vi "L1LeftToCargo7.vi"(9 "Initialized":bool) -> (2 "Drive State":T1)   [LabVIEW 2018]
uses:
  driveStateEnum.ctl
  L1LeftToCargo7.ctl
  driveShifterEnum.ctl
  L1RightToCargo8.ctl
  HatchPanel/hatchPanelEnum.ctl
  HatchPanel/hatchPanelNotifierCluster.ctl
  MotionProfile/Constants.vi
panel:
  out "Speed (ft/s) 3":dbl=5.820510365604576
  in  "Wait til slower then(ft/s) 3":dbl=-3.0
  out "Speed (ft/s) 2":dbl=5.820510365604576
  in  "Wait til slower then(ft/s) 2":dbl=-3.0
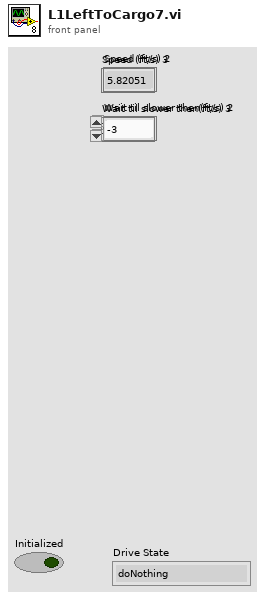
[diagram p1: front panel]
types:
  T1 = typedef "driveStateEnum.ctl" = enum16{"doNothing", "Manuel", "Teleop", "Follow Path (init)", "Follow Path", "Move to Target", "Climb", "Line Align", "Rotate180", "Align50Degrees", "Sonar Brake Tele", "LLCushion", "Auto Approach Target"}
  T2 = typedef "L1LeftToCargo7.ctl" = enum16{"7b -  back away from cargo ship ", "1 - MP move to cargo Ship (init)", "2 - MP move to cargo ship", "3 - Delay for shift", "4 - Approach To Score", "5 - Scored", "99 - doNothing", "7a - back away from cargo ship (init)", "8 - Hatch Panel Motion Off", "9 - Scoring Claw On", "8 - turn towards loading station", "10 - Scoring Claw Off", "11 - MP move towards loading station (init)", "12 -  MP move towards loading station", "13 - MP Move towards  cargo ship *2 (init)", "14 - MP Move towards  cargo ship *2"}
  T3 = typedef "WPI_MotorControlDeviceRef.ctl" = cluster{"DeviceStatus":errorcluster, "Type":T4, "PWM":cluster{"PWM Channel":T5, "DeadBand":T6}, "CAN":cluster{"Device Number":u8, "SetOutput VI Ref":variant, "GetOutput VI Ref":variant, "Enable VI Ref":variant, "Disable VI Ref":variant, "Data":variant}, "Invert":bool, "DIO PWM":cluster{"PWM \"Enable\" Channel":T5, "DIOChannel":T7, "PWM Rate":dbl}}
  T4 = typedef "WPI_MotorControlType.ctl" = enum16{"PWM", "CAN", "DIO PWM"}
  T5 = typedef "FPGA_DIOPWMChannel.ctl" = enum8{"PWM 0", "PWM 1", "PWM 2", "PWM 3", "PWM 4", "PWM 5", "PWM 6", "PWM 7", "PWM 8", "PWM 9", "PWM MXP 0", "PWM MXP 1", "PWM MXP 2", "PWM MXP 3", "PWM MXP 4", "PWM MXP 5", "PWM MXP 6", "PWM MXP 7", "PWM MXP 8", "PWM MXP 9", "Invalid"}
  T6 = typedef "WPI_PWMDeadband.ctl" = cluster{"Name":string, "maxPositivePwm":i32, "minPositivePwm":i32, "centerPwm":i32, "maxNegativePwm":i32, "minNegativePwm":i32, "angularRange":u16}
  T7 = typedef "FPGA_DIOChannel.ctl" = enum8{"DIO 0", "DIO 1", "DIO 2", "DIO 3", "DIO 4", "DIO 5", "DIO 6", "DIO 7", "DIO 8", "DIO 9", "DIO MXP 0", "DIO MXP 1", "DIO MXP 2", "DIO MXP 3", "DIO MXP 4", "DIO MXP 5", "DIO MXP 6", "DIO MXP 7", "DIO MXP 8", "DIO MXP 9", "DIO MXP 10", "DIO MXP 11", "DIO MXP 12", "DIO MXP 13", "DIO MXP 14", "DIO MXP 15", "SPI Port CS1", "SPI Port CS2", "SPI Port CS3", "SPI Port MISO", "SPI Port MOSI", "Invalid"}
  T8 = typedef "L1RightToCargo8.ctl" = enum16{"7b -  back away from cargo ship ", "1 - MP move to cargo Ship (init)", "2 - MP move to cargo ship", "3 - Delay for shift", "4 - Approach To Score", "5 - Scored", "99 - doNothing", "7a - back away from cargo ship (init)", "8 - Hatch Panel Motion Off", "9 - Scoring Claw On", "8 - turn towards loading station", "10 - Scoring Claw Off", "11 - MP move towards loading station (init)", "12 -  MP move towards loading station", "13 - MP Move towards  cargo ship *2 (init)", "14 - MP Move towards  cargo ship *2"}
  T9 = typedef "driveShifterEnum.ctl" = enum16{"Low", "High"}
  T10 = typedef "hatchPanelNotifierCluster.ctl" = cluster{"Hatch Panel State":T11, "Mechanism Motion":bool, "Gathering Claw Motion":bool, "Scoring Claw Motion":bool}
  T11 = typedef "hatchPanelEnum.ctl" = enum16{"do nothing", "State Machine", "Stach Mode", "Climb Mode", "Retracted Closed", "Retracted Open", "Extended Closed", "Extended Open"}
  T12 = typedef "CTRE_PigeonIMU_DeviceRef.ctl" = cluster{"DeviceStatus":errorcluster, "Device Number":u8, "Type":T13, "Device ID":u32, "Handle":u64, "UsageFrame":u32, "Library Path":path}
  T13 = typedef "CTRE_PigeonIMU_ConnectionType.ctl" = u32
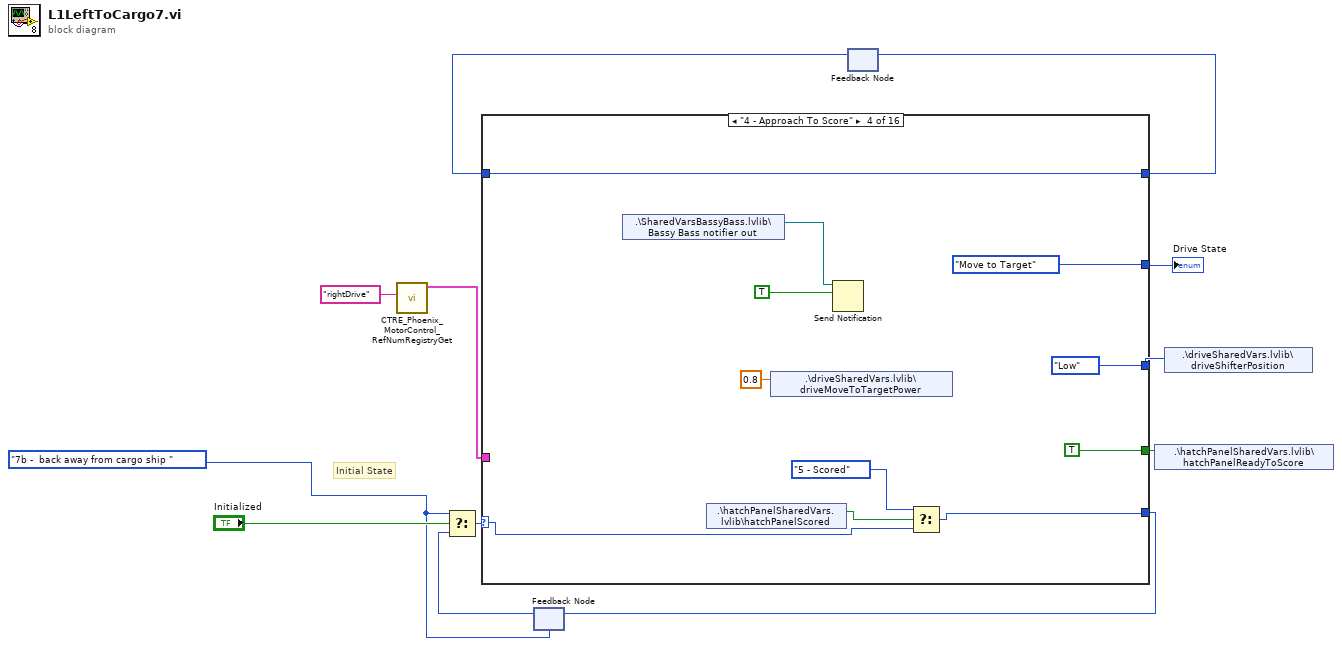
[diagram p0: block diagram]
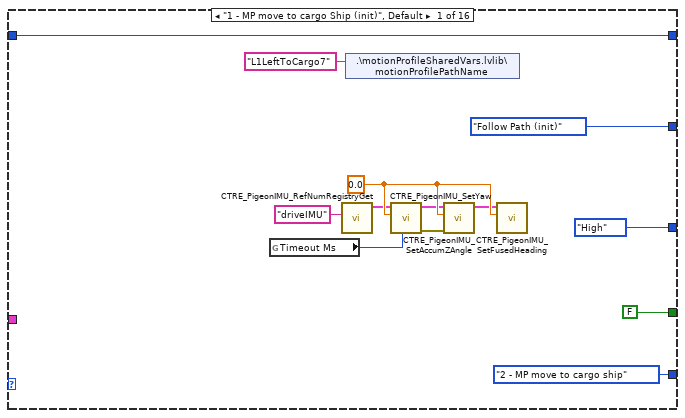
[diagram p2: hidden frame]
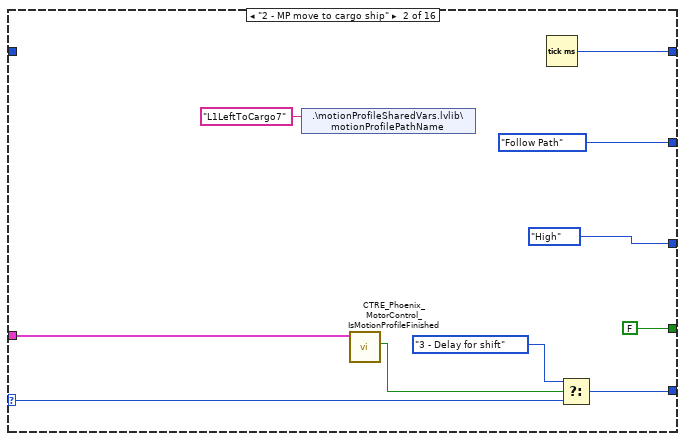
[diagram p3: hidden frame]
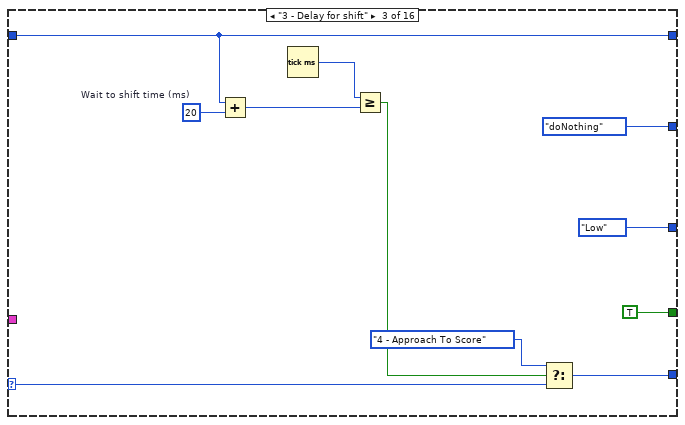
[diagram p4: hidden frame]
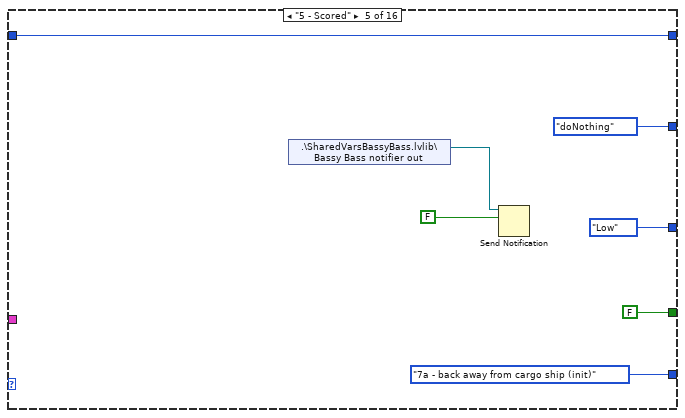
[diagram p5: hidden frame]
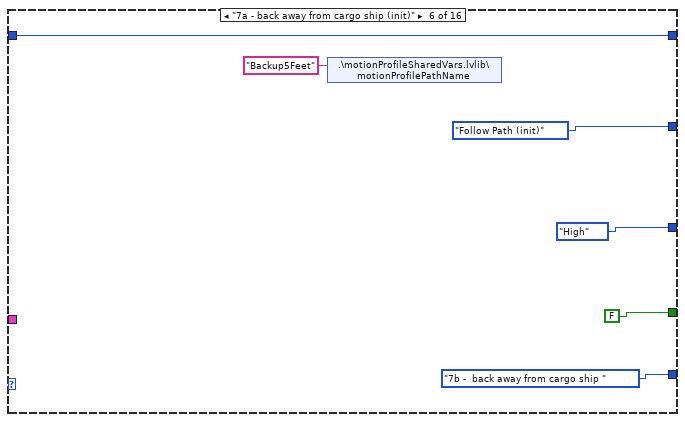
[diagram p6: hidden frame]
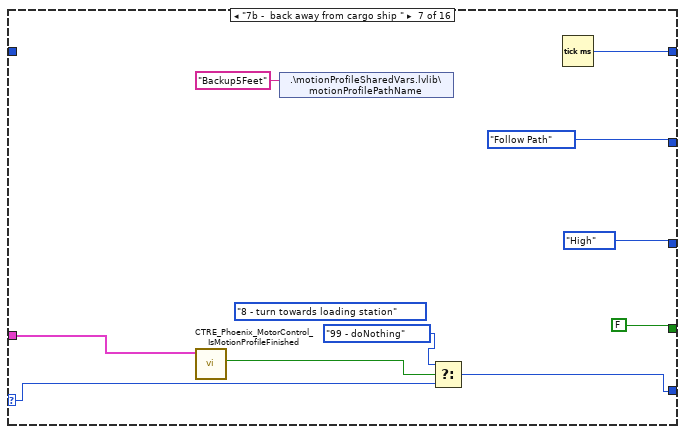
[diagram p7: hidden frame]
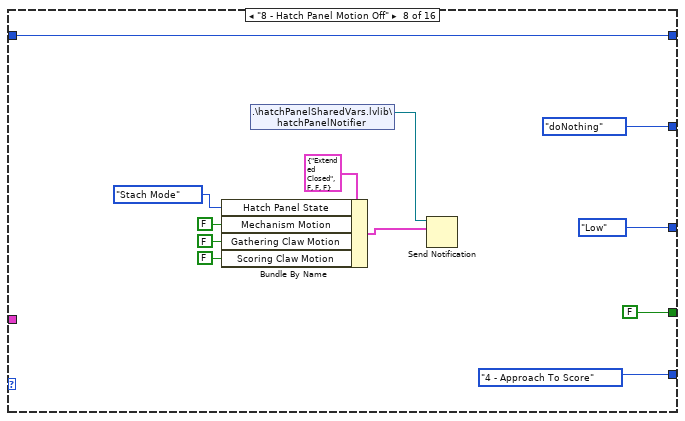
[diagram p8: hidden frame]
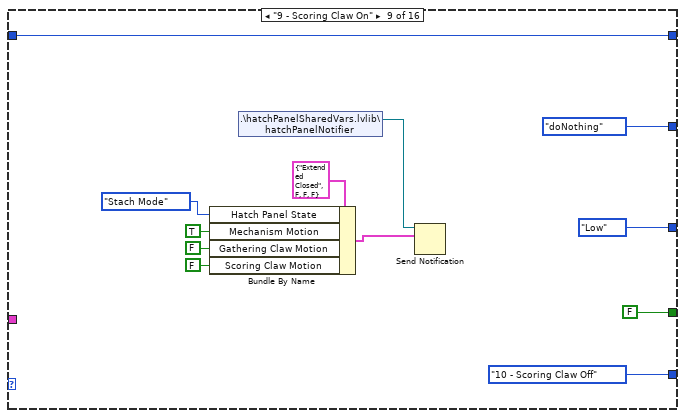
[diagram p9: hidden frame]
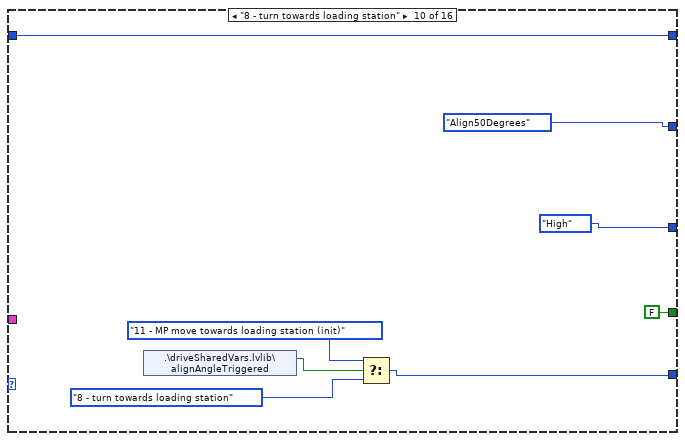
[diagram p10: hidden frame]
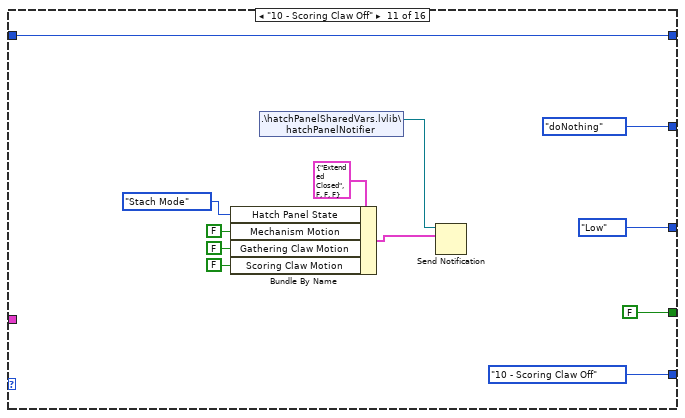
[diagram p11: hidden frame]
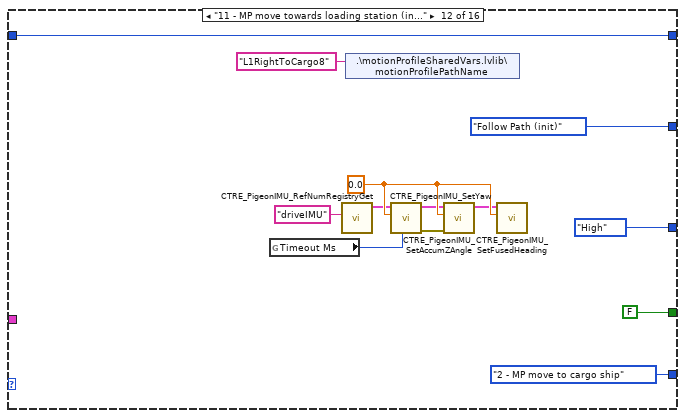
[diagram p12: hidden frame]
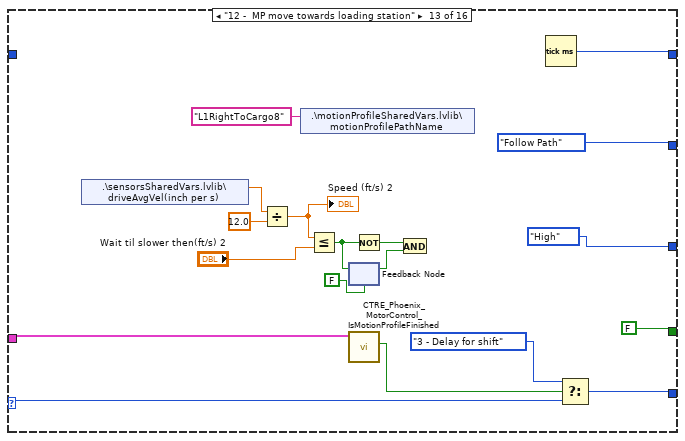
[diagram p13: hidden frame]
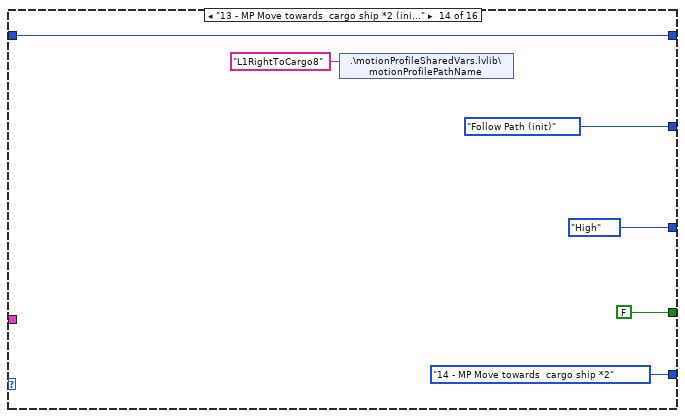
[diagram p14: hidden frame]
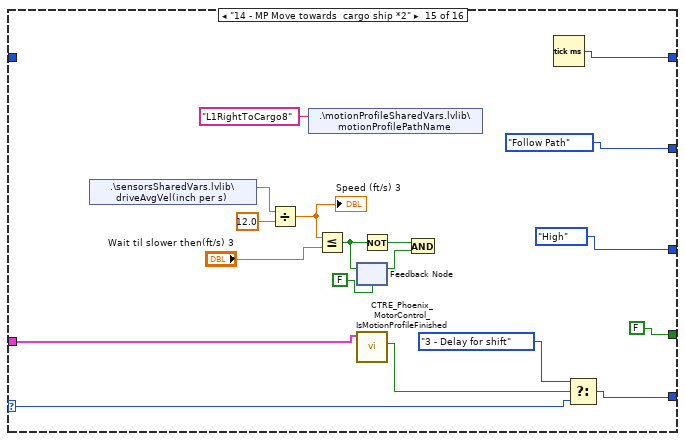
[diagram p15: hidden frame]
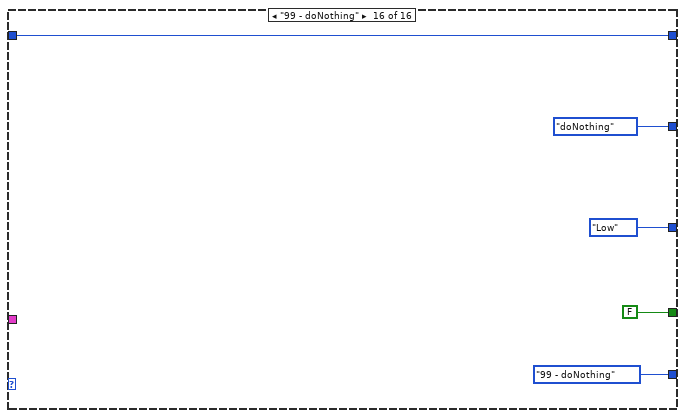
[diagram p16: hidden frame]
diagram:
  w1 = L1LeftToCargo7."7b -  back away from cargo ship " ("Enum")
  # "Initial State"
  n1 = call <vilib>:"CTRE_Phoenix_MotorControl_RefNumRegistryGet.vi"("refnum name"="rightDrive") -> ("PhoenixMotorControlDevRef"=w8:T3)  [unwired: 9 in, 1 out]
  n2 = feedback #1(w1) -> (w11:T8)
  n3 = Select(t=w1, s="Initialized", f=w11) -> (s? t:f=w12:T8)
  n4 = feedback #2() -> (w3:u32)  [unwired: 1 in]
  n5 = case shown="\"4 - Approach To Score\"" w12 {
    selector: w12 -> [_ w33 w38 w51 _ _ w73 _ _ _ _ _ w143 _ w168 _]
    tunnel: [L1RightToCargo8."2 - MP move to cargo ship" ("Enum") w34 w40 w50 L1RightToCargo8."7a - back away from cargo ship (init)" ("Enum") L1RightToCargo8."7b -  back away from cargo ship " ("Enum") w72 L1RightToCargo8."4 - Approach To Score" ("Enum") L1RightToCargo8."10 - Scoring Claw Off" ("Enum") w105 L1RightToCargo8."10 - Scoring Claw Off" ("Enum") L1RightToCargo8."2 - MP move to cargo ship" ("Enum") w144 L1RightToCargo8."14 - MP Move towards  cargo ship *2" ("Enum") w167 L1RightToCargo8."99 - doNothing" ("Enum")] -> w10
    tunnel: [driveStateEnum."Follow Path (init)" ("Drive State Enum") driveStateEnum."Follow Path" ("Drive State Enum") driveStateEnum."doNothing" ("Drive State Enum") driveStateEnum."Move to Target" ("Drive State Enum") driveStateEnum."doNothing" ("Drive State Enum") driveStateEnum."Follow Path (init)" ("Drive State Enum") driveStateEnum."Follow Path" ("Drive State Enum") driveStateEnum."doNothing" ("Drive State Enum") driveStateEnum."doNothing" ("Drive State Enum") driveStateEnum."Align50Degrees" ("Drive State Enum") driveStateEnum."doNothing" ("Drive State Enum") driveStateEnum."Follow Path (init)" ("Drive State Enum") driveStateEnum."Follow Path" ("Drive State Enum") driveStateEnum."Follow Path (init)" ("Drive State Enum") driveStateEnum."Follow Path" ("Drive State Enum") driveStateEnum."doNothing" ("Drive State Enum")] -> w6
    tunnel: w8 -> [_ w31 _ _ _ _ w74 _ _ _ _ _ w142 _ w162 _]
    tunnel: [driveShifterEnum."High" ("driveShifterPosition") driveShifterEnum."High" ("driveShifterPosition") driveShifterEnum."Low" ("driveShifterPosition") driveShifterEnum."Low" ("driveShifterPosition") driveShifterEnum."Low" ("driveShifterPosition") driveShifterEnum."High" ("driveShifterPosition") driveShifterEnum."High" ("driveShifterPosition") driveShifterEnum."Low" ("driveShifterPosition") driveShifterEnum."Low" ("driveShifterPosition") driveShifterEnum."High" ("driveShifterPosition") driveShifterEnum."Low" ("driveShifterPosition") driveShifterEnum."High" ("driveShifterPosition") driveShifterEnum."High" ("driveShifterPosition") driveShifterEnum."High" ("driveShifterPosition") driveShifterEnum."High" ("driveShifterPosition") driveShifterEnum."Low" ("driveShifterPosition")] -> w5
    tunnel: [w15 w28 w44 w55 w60 w69 w75 w85 w97 w111 w114 w126 w139 w160 w163 w180] -> w4
    tunnel: w3 -> [w15 _ w44 w55 w60 w69 _ w85 w97 w111 w114 w126 _ w160 _ w180]
    tunnel: [FALSE FALSE TRUE TRUE FALSE FALSE FALSE FALSE FALSE FALSE FALSE FALSE FALSE FALSE FALSE FALSE] -> w2
    frame "1 - MP move to cargo Ship (init)", Default {
      w23 = 0.0 ("Angle (Deg)")
      n6 = global read "Constants.vi" "Timeout Ms"() -> (w20:i32)
      n7 = call <vilib>:"CTRE_PigeonIMU_RefNumRegistryGet.vi"("refnum name"="driveIMU") -> ("PigeonIMUDevRef"=w17:T12)  [unwired: 9 in, 1 out]
      n8 = shared-variable ".\\motionProfileSharedVars.lvlib\\motionProfilePathName"("L1LeftToCargo7" ("motionProfilePathName")) -> ()  [unwired: 1 in, 1 out]
      n9 = call <vilib>:"CTRE_PigeonIMU_SetYaw.vi"("timeoutMs"=w20, "Value"=w23, "PigeonIMUDevRef"=w17) -> ("error out"=w18:errorcluster, "PigeonIMUDevRef"=w19:T12)  [unwired: 7 in]
      n10 = call <vilib>:"CTRE_PigeonIMU_SetAccumZAngle.vi"("error in (no error)"=w18, "Angle (Deg)"=w23, "PigeonIMUDevRef"=w19) -> ("PigeonIMUDevRef"=w21:T12)  [unwired: 7 in, 1 out]
      n11 = call <vilib>:"CTRE_PigeonIMU_SetFusedHeading.vi"("Value"=w23, "PigeonIMUDevRef 2"=w21) -> ()  [unwired: 8 in, 2 out]
    }
    frame "2 - MP move to cargo ship" {
      n12 = shared-variable ".\\motionProfileSharedVars.lvlib\\motionProfilePathName"("L1LeftToCargo7" ("motionProfilePathName")) -> ()  [unwired: 1 in, 1 out]
      n13 = call <vilib>:"CTRE_Phoenix_MotorControl_IsMotionProfileFinished.vi"("PhoenixMotorControlDevRef"=w31) -> ("Is Motion Profile Finished?"=w30:bool)  [unwired: 8 in, 2 out]
      n14 = Tick Count (ms)() -> (millisecond timer value=w28:u32)
      n15 = Select(t=L1RightToCargo8."3 - Delay for shift", s=w30, f=w33) -> (s? t:f=w34:T8)
    }
    frame "3 - Delay for shift" {
      w43 = u32 20  # Wait to shift time (ms)
      n16 = Add(x=w44, y=w43) -> (x+y=w41:u32)
      n17 = Tick Count (ms)() -> (millisecond timer value=w42:u32)
      n18 = Greater Or Equal?(x=w42, y=w41) -> (x >= y?=w39:bool)
      n19 = Select(t=L1RightToCargo8."4 - Approach To Score", s=w39, f=w38) -> (s? t:f=w40:T8)
    }
    frame "4 - Approach To Score" {
      n20 = shared-variable ".\\SharedVarsBassyBass.lvlib\\Bassy Bass notifier out"() -> (w49:refnum<notifier>)  [unwired: 1 in, 1 out]
      n21 = shared-variable ".\\hatchPanelSharedVars.lvlib\\hatchPanelScored"() -> (w52:bool)  [unwired: 1 in, 1 out]
      n22 = shared-variable ".\\driveSharedVars.lvlib\\driveMoveToTargetPower"(0.8 ("driveMoveToTargetPower")) -> ()  [unwired: 1 in, 1 out]
      n23 = Send Notification(notification=TRUE, notifier=w49) -> ()  [unwired: 1 in, 2 out]
      n24 = Select(t=L1RightToCargo8."5 - Scored", s=w52, f=w51) -> (s? t:f=w50:T8)
    }
    frame "5 - Scored" {
      n25 = shared-variable ".\\SharedVarsBassyBass.lvlib\\Bassy Bass notifier out"() -> (w59:refnum<notifier>)  [unwired: 1 in, 1 out]
      n26 = Send Notification(notification=FALSE, notifier=w59) -> ()  [unwired: 1 in, 2 out]
    }
    frame "7a - back away from cargo ship (init)" {
      n27 = shared-variable ".\\motionProfileSharedVars.lvlib\\motionProfilePathName"("Backup5Feet" ("motionProfilePathName")) -> ()  [unwired: 1 in, 1 out]
    }
    frame "7b -  back away from cargo ship " {
      (unwired) L1RightToCargo8."8 - turn towards loading station" ("t")
      n28 = call <vilib>:"CTRE_Phoenix_MotorControl_IsMotionProfileFinished.vi"("PhoenixMotorControlDevRef"=w74) -> ("Is Motion Profile Finished?"=w77:bool)  [unwired: 8 in, 2 out]
      n29 = shared-variable ".\\motionProfileSharedVars.lvlib\\motionProfilePathName"("Backup5Feet" ("motionProfilePathName")) -> ()  [unwired: 1 in, 1 out]
      n30 = Select(t=L1RightToCargo8."99 - doNothing", s=w77, f=w73) -> (s? t:f=w72:T8)
      n31 = Tick Count (ms)() -> (millisecond timer value=w75:u32)
    }
    frame "8 - Hatch Panel Motion Off" {
      n32 = Bundle By Name(cluster=T10 {"Hatch Panel State"=enum."Extended Closed", "Mechanism Motion"=FALSE, "Gathering Claw Motion"=FALSE, "Scoring Claw Motion"=FALSE} ("notification"), "Hatch Panel State"=hatchPanelEnum."Stach Mode", "Mechanism Motion"=FALSE, "Gathering Claw Motion"=FALSE, "Scoring Claw Motion"=FALSE) -> (w89:T10)
      n33 = shared-variable ".\\hatchPanelSharedVars.lvlib\\hatchPanelNotifier"() -> (w90:refnum<notifier>)  [unwired: 1 in, 1 out]
      n34 = Send Notification(notification=w89, notifier=w90) -> ()  [unwired: 1 in, 2 out]
    }
    frame "9 - Scoring Claw On" {
      n35 = Bundle By Name(cluster=T10 {"Hatch Panel State"=enum."Extended Closed", "Mechanism Motion"=FALSE, "Gathering Claw Motion"=FALSE, "Scoring Claw Motion"=FALSE} ("notification"), "Hatch Panel State"=hatchPanelEnum."Stach Mode", "Mechanism Motion"=TRUE, "Gathering Claw Motion"=FALSE, "Scoring Claw Motion"=FALSE) -> (w101:T10)
      n36 = shared-variable ".\\hatchPanelSharedVars.lvlib\\hatchPanelNotifier"() -> (w102:refnum<notifier>)  [unwired: 1 in, 1 out]
      n37 = Send Notification(notification=w101, notifier=w102) -> ()  [unwired: 1 in, 2 out]
    }
    frame "8 - turn towards loading station" {
      n38 = shared-variable ".\\driveSharedVars.lvlib\\alignAngleTriggered"() -> (w108:bool)  [unwired: 1 in, 1 out]
      n39 = Select(t=L1RightToCargo8."11 - MP move towards loading station (init)" ("Enum"), s=w108, f=L1RightToCargo8."8 - turn towards loading station" ("Enum")) -> (s? t:f=w105:T8)
    }
    frame "10 - Scoring Claw Off" {
      n40 = Bundle By Name(cluster=T10 {"Hatch Panel State"=enum."Extended Closed", "Mechanism Motion"=FALSE, "Gathering Claw Motion"=FALSE, "Scoring Claw Motion"=FALSE} ("notification"), "Hatch Panel State"=hatchPanelEnum."Stach Mode", "Mechanism Motion"=FALSE, "Gathering Claw Motion"=FALSE, "Scoring Claw Motion"=FALSE) -> (w121:T10)
      n41 = shared-variable ".\\hatchPanelSharedVars.lvlib\\hatchPanelNotifier"() -> (w122:refnum<notifier>)  [unwired: 1 in, 1 out]
      n42 = Send Notification(notification=w121, notifier=w122) -> ()  [unwired: 1 in, 2 out]
    }
    frame "11 - MP move towards loading station (init)" {
      w135 = 0.0 ("Angle (Deg)")
      n43 = global read "Constants.vi" "Timeout Ms"() -> (w132:i32)
      n44 = call <vilib>:"CTRE_PigeonIMU_RefNumRegistryGet.vi"("refnum name"="driveIMU") -> ("PigeonIMUDevRef"=w129:T12)  [unwired: 9 in, 1 out]
      n45 = shared-variable ".\\motionProfileSharedVars.lvlib\\motionProfilePathName"("L1RightToCargo8" ("motionProfilePathName")) -> ()  [unwired: 1 in, 1 out]
      n46 = call <vilib>:"CTRE_PigeonIMU_SetYaw.vi"("timeoutMs"=w132, "Value"=w135, "PigeonIMUDevRef"=w129) -> ("error out"=w130:errorcluster, "PigeonIMUDevRef"=w131:T12)  [unwired: 7 in]
      n47 = call <vilib>:"CTRE_PigeonIMU_SetAccumZAngle.vi"("error in (no error)"=w130, "Angle (Deg)"=w135, "PigeonIMUDevRef"=w131) -> ("PigeonIMUDevRef"=w133:T12)  [unwired: 7 in, 1 out]
      n48 = call <vilib>:"CTRE_PigeonIMU_SetFusedHeading.vi"("Value"=w135, "PigeonIMUDevRef 2"=w133) -> ()  [unwired: 8 in, 2 out]
    }
    frame "12 -  MP move towards loading station" {
      n49 = shared-variable ".\\sensorsSharedVars.lvlib\\driveAvgVel(inch per s)"() -> (w149:dbl)  [unwired: 1 in, 1 out]
      n50 = Divide(x=w149, y=12.0) -> (x/y=w150:dbl)
      "Speed (ft/s) 2" <- w150
      n51 = shared-variable ".\\motionProfileSharedVars.lvlib\\motionProfilePathName"("L1RightToCargo8" ("motionProfilePathName")) -> ()  [unwired: 1 in, 1 out]
      n52 = Less Or Equal?(x=w150, y="Wait til slower then(ft/s) 2") -> (x <= y?=w152:bool)
      n53 = feedback #3(FALSE) -> (w153:bool)
      n54 = feedback-in #3(w152) -> ()
      n55 = call <vilib>:"CTRE_Phoenix_MotorControl_IsMotionProfileFinished.vi"("PhoenixMotorControlDevRef"=w142) -> ("Is Motion Profile Finished?"=w155:bool)  [unwired: 8 in, 2 out]
      n56 = Not(x=w152) -> (.not. x?=w154:bool)
      n57 = And(x=w154, y=w153) -> ()  [unwired: 1 out]
      n58 = Tick Count (ms)() -> (millisecond timer value=w139:u32)
      n59 = Select(t=L1RightToCargo8."3 - Delay for shift", s=w155, f=w143) -> (s? t:f=w144:T8)
    }
    frame "13 - MP Move towards  cargo ship *2 (init)" {
      n60 = shared-variable ".\\motionProfileSharedVars.lvlib\\motionProfilePathName"("L1RightToCargo8" ("motionProfilePathName")) -> ()  [unwired: 1 in, 1 out]
    }
    frame "14 - MP Move towards  cargo ship *2" {
      n61 = shared-variable ".\\sensorsSharedVars.lvlib\\driveAvgVel(inch per s)"() -> (w173:dbl)  [unwired: 1 in, 1 out]
      n62 = Divide(x=w173, y=12.0) -> (x/y=w174:dbl)
      "Speed (ft/s) 3" <- w174
      n63 = shared-variable ".\\motionProfileSharedVars.lvlib\\motionProfilePathName"("L1RightToCargo8" ("motionProfilePathName")) -> ()  [unwired: 1 in, 1 out]
      n64 = Less Or Equal?(x=w174, y="Wait til slower then(ft/s) 3") -> (x <= y?=w176:bool)
      n65 = feedback #4(FALSE) -> (w177:bool)
      n66 = feedback-in #4(w176) -> ()
      n67 = call <vilib>:"CTRE_Phoenix_MotorControl_IsMotionProfileFinished.vi"("PhoenixMotorControlDevRef"=w162) -> ("Is Motion Profile Finished?"=w179:bool)  [unwired: 8 in, 2 out]
      n68 = Not(x=w176) -> (.not. x?=w178:bool)
      n69 = And(x=w178, y=w177) -> ()  [unwired: 1 out]
      n70 = Tick Count (ms)() -> (millisecond timer value=w163:u32)
      n71 = Select(t=L1RightToCargo8."3 - Delay for shift", s=w179, f=w168) -> (s? t:f=w167:T8)
    }
    frame "99 - doNothing" {
    }
  }
  "Drive State" <- w6
  n72 = feedback-in #1(w10) -> ()
  n73 = feedback-in #2(w4) -> ()
  n74 = shared-variable ".\\hatchPanelSharedVars.lvlib\\hatchPanelReadyToScore"(w2) -> ()  [unwired: 1 in, 1 out]
  n75 = shared-variable ".\\driveSharedVars.lvlib\\driveShifterPosition"(w5) -> ()  [unwired: 1 in, 1 out]
